vi "Get Res_Attendance.vi"(8 "error in (no error)":errorcluster, 11 "AttendRecord in":refnum<class "AttendRecord.lvclass">) -> (0 "error out":errorcluster, 1 "NumOfAttendance":T1, 2 "Res_Attendance":cluster{"BackGround":u32, "Reason":string}[][](array[cluster]), 3 "AttendRecord out":refnum<class "AttendRecord.lvclass">)   [LabVIEW 2015, in "Admin_Actor.lvlib" / "AttendRecord.lvclass"]
uses:
  AttendRecord.lvclass
  CalAttendance/Type Definitions/NumOfAttendace.ctl
  AttendRecord.lvclass/AttendRecord.ctl
  CalAttendance/CalAttendance.lvclass
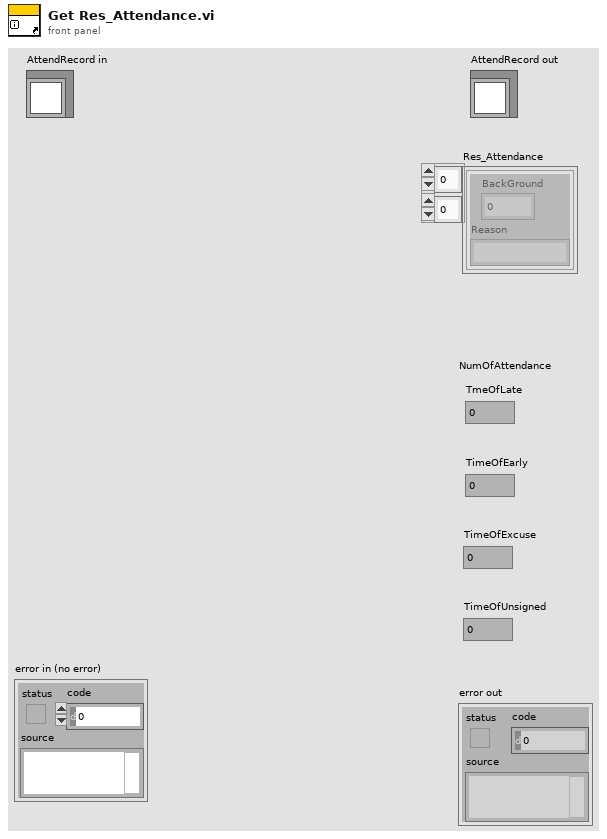
[diagram p1: front panel]
types:
  T1 = typedef "Admin_Actor.lvlib/CalAttendance.lvclass/NumOfAttendace.ctl" = cluster{"TmeOfLate":i32, "TimeOfEarly":i32, "TimeOfExcuse":i32, "TimeOfUnsigned":i32}
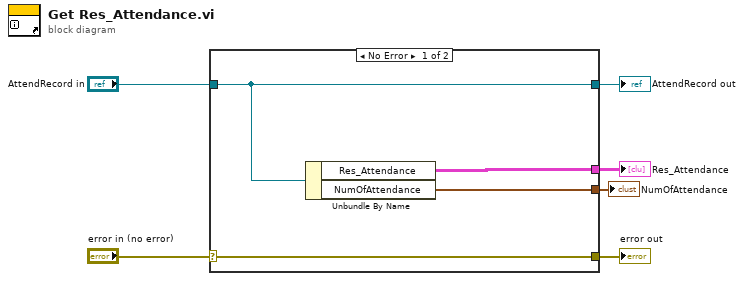
[diagram p0: block diagram]
diagram:
  n1 = case shown="No Error" "error in (no error)" {
    selector: "error in (no error)" -> [w10 w11]
    tunnel: [w10 w11] -> w5
    tunnel: [w9 w12] -> w3
    tunnel: "AttendRecord in" -> [w9 w12]
    tunnel: [w8 _] -> w2
    tunnel: [w7 _] -> w1
    frame No Error {
      n2 = Unbundle By Name(w9) -> ("Res_Attendance"=w8:cluster{"BackGround":u32, "Reason":string}[][], "NumOfAttendance"=w7:T1)
    }
    frame Error {
    }
  }
  "error out" <- w5
  "AttendRecord out" <- w3
  "Res_Attendance" <- w2
  "NumOfAttendance" <- w1
